vi "Check if fit can be placed in stream array.vi"(10 "Fit Number":i32, 11 "Stream Array":T1[](array[typedef])) -> (1 "Possible Out":bool, 3 "Remaining Stream Out":T1[](array[typedef]))   [LabVIEW 2023]
uses:
  ENUM_Type.ctl
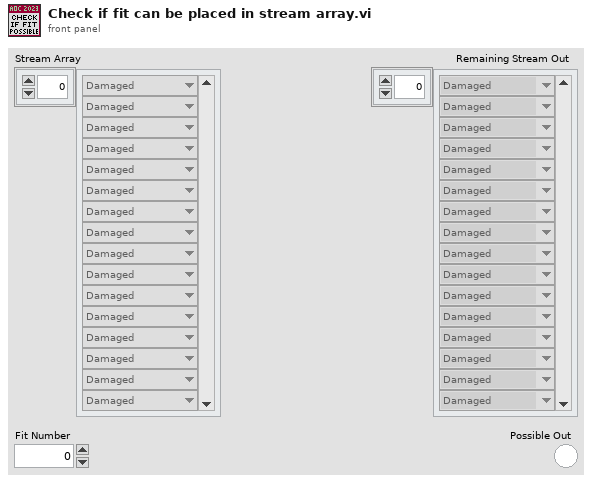
[diagram p1: front panel]
types:
  T1 = typedef "ENUM_Type.ctl" = enum16{"Damaged", "Operational", "Unknown"}
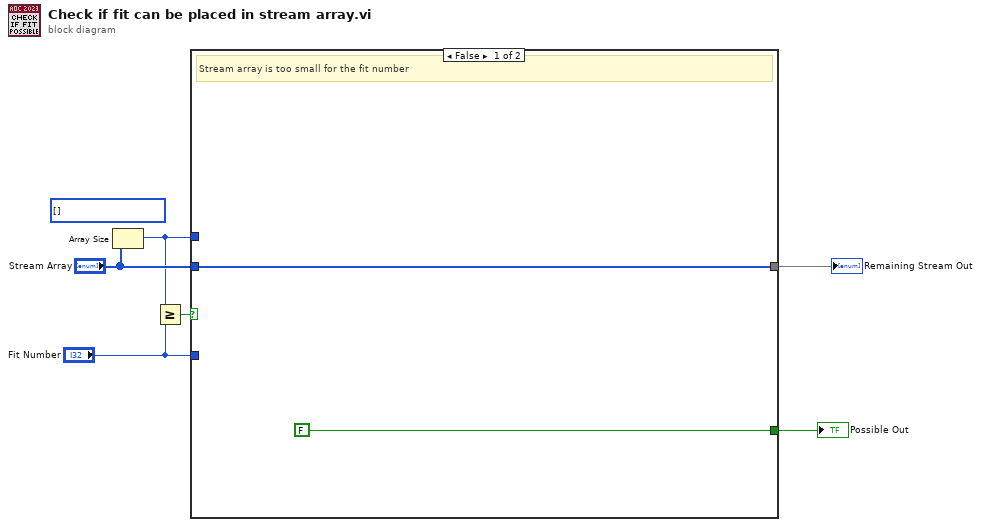
[diagram p0: block diagram]
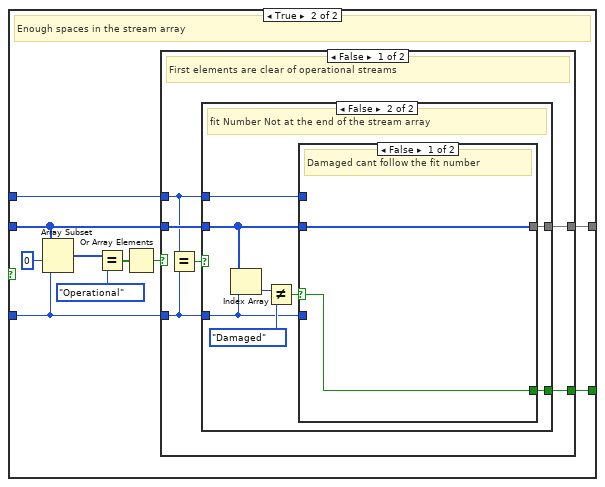
[diagram p2: hidden frame]
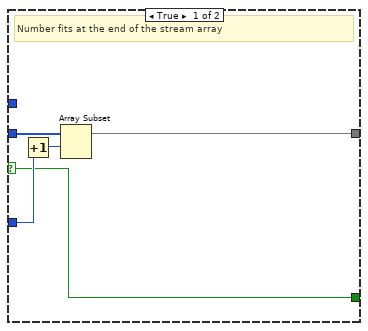
[diagram p3: hidden frame]
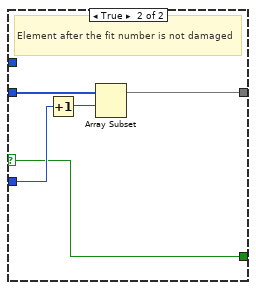
[diagram p4: hidden frame]
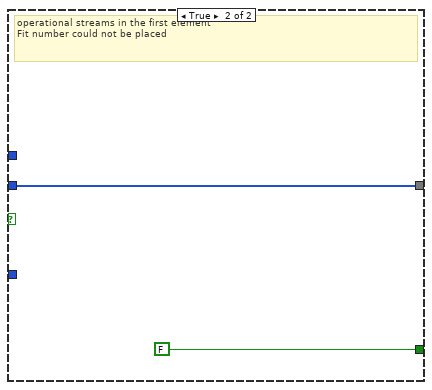
[diagram p5: hidden frame]
diagram:
  (unwired) T1[] [] items=["Damaged", "Operational", "Unknown"] ("Stream Array")
  n1 = Array Size(array="Stream Array") -> (size(s)=w3:i32)
  n2 = Greater Or Equal?(x=w3, y="Fit Number") -> (x >= y?=w6:bool)
  n3 = case shown="False" w6 {
    tunnel: "Stream Array" -> [w8 w13]
    tunnel: "Fit Number" -> [_ w12]
    tunnel: w3 -> [_ w14]
    tunnel: [w8 w10] -> w2
    tunnel: [FALSE w9] -> w1
    frame False {
      # "Stream array is too small for the fit number"
    }
    frame True {
      # "Enough spaces in the stream array"
      n4 = Array Subset(array=w13, index=0, length=w12) -> (w18:T1[])
      n5 = Equal?(x=w18, y=ENUM_Type."Operational" ("Enum")) -> (x = y?=w16:bool[])
      n6 = Or Array Elements(Boolean array=w16) -> (logical OR=w15:bool)
      n7 = case shown="False" w15 {
        tunnel: w14 -> [w22 _]
        tunnel: w13 -> [w24 w46]
        tunnel: w12 -> [w21 _]
        tunnel: [w23 w46] -> w10
        tunnel: [w19 FALSE] -> w9
        frame False {
          # "First elements are clear of operational streams"
          n8 = Equal?(x=w22, y=w21) -> (x = y?=w20:bool)
          n9 = case shown="False" w20 {
            selector: w20 -> [w25 _]
            tunnel: w22 -> [_ w34]
            tunnel: w24 -> [w29 w33]
            tunnel: w21 -> [w28 w32]
            tunnel: [w27 w31] -> w23
            tunnel: [w25 w30] -> w19
            frame True {
              # "Number fits at the end of the stream array"
              n10 = Increment(x=w28) -> (x+1=w26:i32)
              n11 = Array Subset(array=w29, index=w26) -> (w27:T1[])  [unwired: 1 in]
            }
            frame False {
              # "fit Number Not at the end of the stream array"
              n12 = Index Array(array=w33, index=w32) -> (element=w37:T1)
              n13 = Not Equal?(x=w37, y=ENUM_Type."Damaged") -> (x != y?=w35:bool)
              n14 = case shown="False" w35 {
                selector: w35 -> [w39 w40]
                tunnel: w34 -> [_ _]
                tunnel: w33 -> [w38 w44]
                tunnel: w32 -> [_ w43]
                tunnel: [w38 w41] -> w31
                tunnel: [w39 w40] -> w30
                frame False {
                  # "Damaged cant follow the fit number"
                }
                frame True {
                  # "Element after the fit number is not damaged"
                  n15 = Increment(x=w43) -> (x+1=w42:i32)
                  n16 = Array Subset(array=w44, index=w42) -> (w41:T1[])  [unwired: 1 in]
                }
              }
            }
          }
        }
        frame True {
          # "operational streams in the first element\nFit number could not be placed"
        }
      }
    }
  }
  "Possible Out" <- w1
  "Remaining Stream Out" <- w2
